vi "总磷总氮版本号读取.vi"(8 "Error in":errorcluster caption="Error in (no error)", 11 "MB session in":refnum<class "MB_Master.lvclass">) -> (0 "error out":errorcluster, 2 "固件版本号":string, 3 "MB session out":refnum<class "MB_Master.lvclass">)   [LabVIEW 2016, in "斯坦道氨氮.lvlib"]
uses:
  <vilib>/Plasmionique/MB Master/MB_Master/MB_Master.lvclass
  <vilib>/Plasmionique/MB Master/MB Master.lvlib
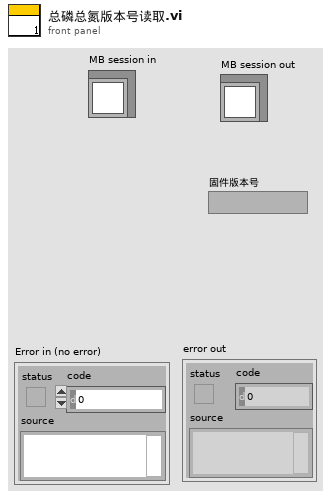
[diagram p1: front panel]
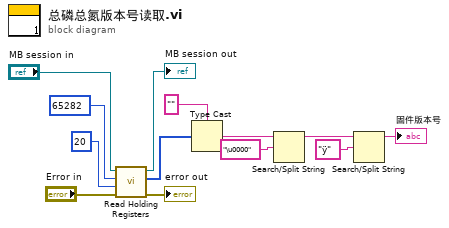
[diagram p0: block diagram]
diagram:
  n1 = call <vilib>:"Read Holding Registers.vi"("error in (no error)"="Error in", "quantity"=u16 20, "starting address"=u16 65282, "MB session in"="MB session in") -> ("error out"=→"error out":errorcluster, "Registers"=w5:u16[], "MB session out"=→"MB session out":refnum<class "MB_Master.lvclass">)  [unwired: 5 in]
  n2 = Type Cast(type="", x=w5) -> (*(type *) &x=w4:string)
  n3 = Search/Split String(string=w4, search string/char (-)="\u0000" ("搜索字符串")) -> (substring before match=w3:string)  [unwired: 1 in, 2 out]
  n4 = Search/Split String(string=w3, search string/char (-)="ÿ" ("搜索字符串")) -> (substring before match=→"固件版本号":string)  [unwired: 1 in, 2 out]
